vi "Set Listbox Position.vi"(5 "Visible?":bool, 7 "Multicolumn Listbox":refnum<vi>, 8 "error in (no error)":errorcluster, 10 "Active Cell":cluster{"Row":i32, "Column":i32}, 11 "Popup Listbox":refnum<vi>) -> (0 "error out":errorcluster)   [LabVIEW 2012]
uses:
  Property/Get Active Cell Position.vi
  Mlistbox Tools.lvlib
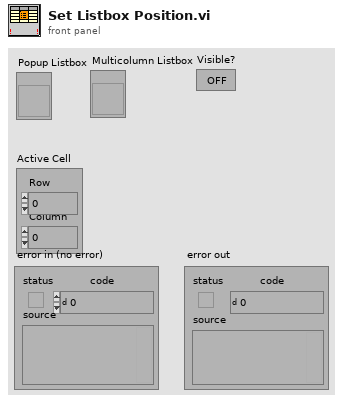
[diagram p1: front panel]
types:
  T1 = typedef "LVPositionTypeDef.ctl" = cluster{"Left":i32, "Top":i32}
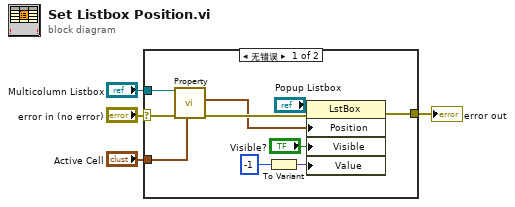
[diagram p0: block diagram]
diagram:
  n1 = case shown="无错误" "error in (no error)" {
    selector: "error in (no error)" -> [w8 w15]
    tunnel: [w12 w15] -> w3
    tunnel: "Multicolumn Listbox" -> [w9 _]
    tunnel: "Active Cell" -> [w7 _]
    frame No Error {
      n2 = call-poly "Property.vi"("Active Cell In"=w7, "错误输入"=w8, "Mlistbox Ref"=w9) -> ("错误输出"=w6:errorcluster, "CellPos Out"=w5:T1)  [unwired: 6 in, 1 out]
      n3 = To Variant(anything=-1) -> (Variant=w11:variant)
      n4 = property class="LstBox"(reference="Popup Listbox", error in=w6, "Position"=w5, "Visible"="Visible?", "Value"=w11) -> (error out=w12:errorcluster)  [unwired: 1 out]
    }
    frame Error {
    }
  }
  "error out" <- w3
